vi "Connect.vi"(8 "error in (no error)":errorcluster, 11 "Statnett C37.118 DLL in":refnum<class "Statnett C37.118 DLL.lvclass">) -> (0 "error out":errorcluster, 3 "Statnett C37.118 DLL out":refnum<class "Statnett C37.118 DLL.lvclass">)   [LabVIEW 2013, in "PMU Recorder Light.lvlib" / "Statnett C37.118 DLL.lvclass"]
uses:
  Statnett C37.118 DLL.lvclass
  Statnett C37.118 DLL.lvclass/Statnett C37.118 DLL.ctl
  c37118-dll/C37118-DLL.lvlib
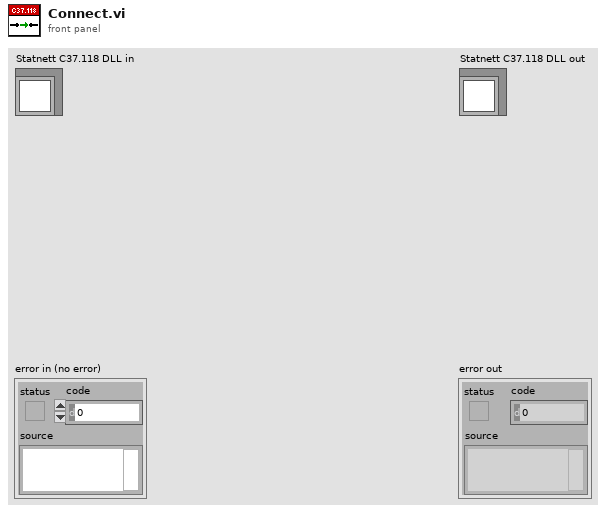
[diagram p1: front panel]
types:
  T1 = cluster{"IP-address":string, "Port":string, "ID Code":u32}
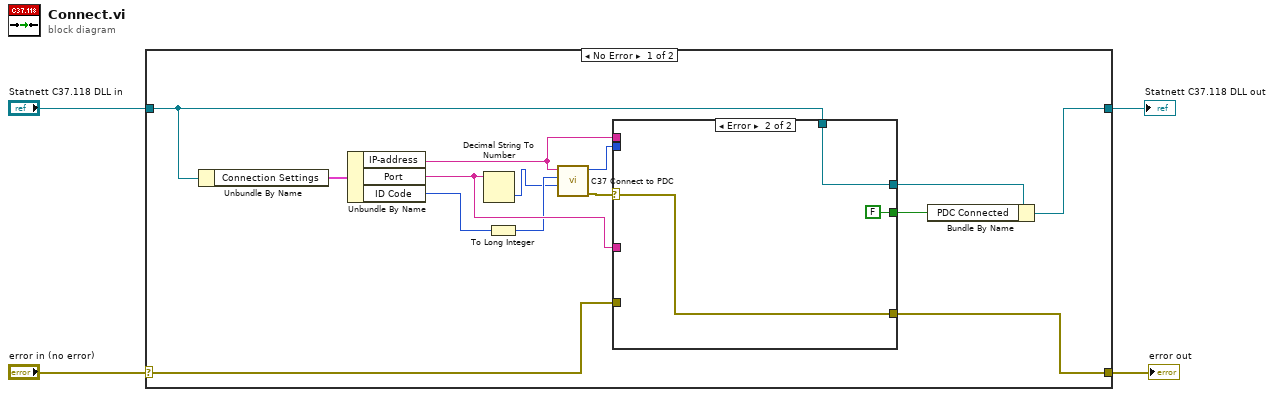
[diagram p0: block diagram]
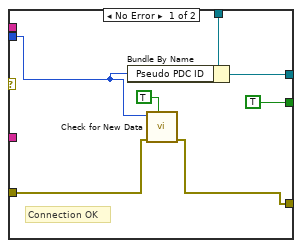
[diagram p2: hidden frame]
diagram:
  n1 = case shown="No Error" "error in (no error)" {
    selector: "error in (no error)" -> [w15 w30]
    tunnel: [w14 w30] -> w3
    tunnel: [w10 w29] -> w1
    tunnel: "Statnett C37.118 DLL in" -> [w16 w29]
    frame No Error {
      n2 = Unbundle By Name(w16) -> ("Connection Settings"=w18:T1)
      n3 = Unbundle By Name(w18) -> ("IP-address"=w9:string, "Port"=w13:string, "ID Code"=w17:u32)
      n4 = Decimal String To Number(string=w13) -> (number=w7:i32)  [unwired: 2 in, 1 out]
      n5 = To Long Integer(number=w17) -> (32bit integer=w8:i32)
      n6 = call "C37 Connect to PDC.vi"("Port"=w7, "PDC ID"=w8, "IP Address"=w9) -> ("error out"=w6:errorcluster, "Pseudo PDC ID"=w5:i32)  [unwired: 7 in]
      n7 = case shown="Error" w6 {
        selector: w6 -> [_ w26]
        tunnel: w16 -> [w25 w28]
        tunnel: w5 -> [w19 _]
        tunnel: [w24 w28] -> w11
        tunnel: w15 -> [w22 _]
        tunnel: [w21 w26] -> w14
        tunnel: w9 -> [_ _]
        tunnel: w13 -> [_ _]
        tunnel: [TRUE ("PDC Connected") FALSE ("PDC Connected")] -> w12
        frame No Error {
          # "Connection OK"
          n8 = Bundle By Name(cluster=w25, "Pseudo PDC ID"=w19) -> (w24:refnum<class "Statnett C37.118 DLL.lvclass">)
          n9 = call "Check for New Data.vi"("Set Pseudo PDC ID"=TRUE ("Initialize"), "error in (no error)"=w22, "Pseudo PDC ID"=w19) -> ("error out"=w21:errorcluster)  [unwired: 7 in, 1 out]
        }
        frame Error {
        }
      }
      n10 = Bundle By Name(cluster=w11, "PDC Connected"=w12) -> (w10:refnum<class "Statnett C37.118 DLL.lvclass">)
    }
    frame Error {
    }
  }
  "error out" <- w3
  "Statnett C37.118 DLL out" <- w1
